vi "config CANcoder.vi"(8 "error in (no error)":errorcluster, 9 "SensorCoefficient":dbl, 11 "CANcoder init data":T1) -> (0 "error out":errorcluster)   [LabVIEW 2023]
uses:
  ctrl defs/ctrl CANcoder.ctl
  <vilib>/Rock Robotics/WPI/ThirdParty/Phoenix-LabVIEW/CANCoder/Controls/CTRE_Phoenix_CANcoder_Configurables.ctl
  <vilib>/Rock Robotics/WPI/ThirdParty/Phoenix-LabVIEW/CANCoder/Controls/CTRE_Phoenix_CANcoder_SensorInitializationStrategy.ctl
  <vilib>/Rock Robotics/WPI/ThirdParty/Phoenix-LabVIEW/CANCoder/Controls/CTRE_Phoenix_CANcoder_AbsoluteSensorRange.ctl
  <vilib>/Rock Robotics/WPI/ThirdParty/Phoenix-LabVIEW/Motor Controller/Controls/CTRE_Phoenix_MotorControl_VelocityMeasurementPeriod.ctl
  <vilib>/Rock Robotics/WPI/ThirdParty/Phoenix-LabVIEW/CANCoder/Controls/CTRE_Phoenix_CANcoder_SensorTimeBase.ctl
  <vilib>/Rock Robotics/WPI/ThirdParty/Phoenix-LabVIEW/CANCoder/Set/CTRE_Phoenix_CANcoder_SetPositionToAbsolute.vi
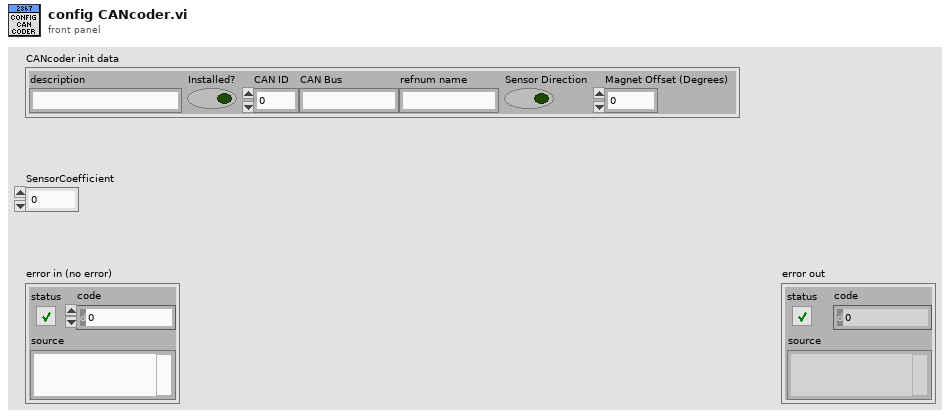
[diagram p1: front panel]
types:
  T1 = typedef "ctrl CANcoder.ctl" = cluster{"description":string, "Installed?":bool, "CAN ID":u8, "CAN Bus":string, "refnum name":string, "Sensor Direction":bool, "Magnet Offset (Degrees)":dbl}
  T2 = typedef "CTRE_Phoenix_CANcoder_Configurables.ctl" = cluster{"Sensor Initialization Strategy":T3, "Absolute Sensor Range":T4, "Velocity Measurement Period":T5, "Velocity Measurement Window":i32, "Magnet Offset (Degrees)":dbl, "Sensor Direction":bool, "Sensor Coefficient":dbl, "Unit String":string, "Sensor Time Base":T6}
  T3 = typedef "CTRE_Phoenix_CANcoder_SensorInitializationStrategy.ctl" = enum16{"Boot To Zero", "Boot To Absolute Position"}
  T4 = typedef "CTRE_Phoenix_CANcoder_AbsoluteSensorRange.ctl" = enum16{"Unsigned [0 to 360)", "Signed [-180 to +180)"}
  T5 = typedef "CTRE_Phoenix_MotorControl_VelocityMeasurementPeriod.ctl" = u16
  T6 = typedef "CTRE_Phoenix_CANcoder_SensorTimeBase.ctl" = enum16{"Per100Ms_Legacy", "PerSecond", "PerMinute"}
  T7 = typedef "CTRE_Phoenix_CANcoder_DeviceRef.ctl" = cluster{"DeviceStatus":errorcluster, "Device Number":u8, "Handle":u64, "UsageFrame":u32, "Library Path":path}
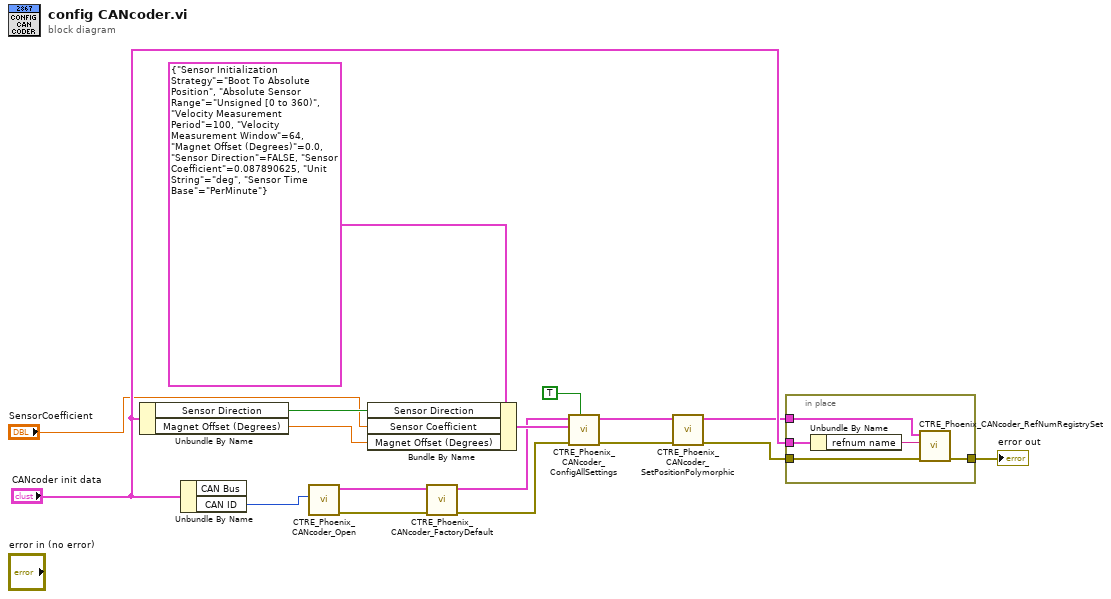
[diagram p0: block diagram]
diagram:
  n1 = Unbundle By Name("CANcoder init data") -> ("Sensor Direction"=w9:bool, "Magnet Offset (Degrees)"=w7:dbl)
  n2 = Unbundle By Name("CANcoder init data") -> ("CAN ID"=w16:u8)  [unwired: 1 out]
  n3 = call <vilib>:"CTRE_Phoenix_CANcoder_Open.vi"("Device Number"=w16) -> ("error out"=w15:errorcluster, "CTRE_CANcoder_DeviceRef"=w17:T7)  [unwired: 9 in]
  n4 = Bundle By Name(cluster=T2 {"Sensor Initialization Strategy"=enum."Boot To Absolute Position", "Absolute Sensor Range"=enum."Unsigned [0 to 360)", "Velocity Measurement Period"=100, "Velocity Measurement Window"=64, "Magnet Offset (Degrees)"=0.0, "Sensor Direction"=FALSE, "Sensor Coefficient"=0.087890625, "Unit String"="deg", "Sensor Time Base"=enum."PerMinute"} ("CANcoder Configurables"), "Sensor Direction"=w9, "Sensor Coefficient"="SensorCoefficient", "Magnet Offset (Degrees)"=w7) -> (w10:T2)
  n5 = call <vilib>:"CTRE_Phoenix_CANcoder_FactoryDefault.vi"("error in"=w15, "CTRE_CANcoder_DeviceRef"=w17) -> ("error out"=w5:errorcluster, "CTRE_CANcoder_DeviceRef"=w6:T7)  [unwired: 8 in]
  n6 = call <vilib>:"CTRE_Phoenix_CANcoder_ConfigAllSettings.vi"("Force Write"=TRUE, "error in (no error)"=w5, "CANcoder Configurables"=w10, "CTRE_CANcoder_DeviceRef"=w6) -> ("error out"=w3:errorcluster, "CTRE_CANcoder_DeviceRef"=w4:T7)  [unwired: 6 in]
  n7 = call-poly <vilib>:"CTRE_Phoenix_CANcoder_SetPositionPolymorphic.vi"("error in (no error)"=w3, "CTRE_CANcoder_DeviceRef"=w4) -> ("error out"=w1:errorcluster, "CTRE_CANcoder_DeviceRef"=w2:T7)  [unwired: 8 in]
  n8 = in-place {
    in-place-border: [w21] -> w14
    in-place-border: "CANcoder init data" -> [w20]
    in-place-border: w2 -> [w19]
    in-place-border: w1 -> [w18]
    n9 = Unbundle By Name(w20) -> ("refnum name"=w22:string)
    n10 = call <vilib>:"CTRE_Phoenix_CANcoder_RefNumRegistrySet.vi"("error in (no error)"=w18, "refnum name"=w22, "CTRE_CANcoder_DeviceRef"=w19) -> ("error out"=w21:errorcluster)  [unwired: 7 in, 1 out]
  }
  "error out" <- w14
